vi "fit voltage data to line.vi"(0 "display queues":T1, 1 "disk queues":T1, 5 "crossing time":dbl, 7 "new crossing":bool, 9 "time_buffer":dbl=0.15, 11 "error in (no error)":errorcluster) -> (4 "slope":dbl, 6 "graph":cluster{dbl[], "Best Linear Fit":dbl[]}, 15 "error out":errorcluster)   [LabVIEW 2017]
uses:
  typedefs/queue cluster.ctl
  typedefs/reading queue.ctl
  typedefs/reading.ctl
  typedefs/readingType.ctl
  typedefs/reading1.ctl
  <vilib>/Analysis/6fits.llb/Curve Fitting Criteria.ctl
  <vilib>/Analysis/NI_AALPro.lvlib
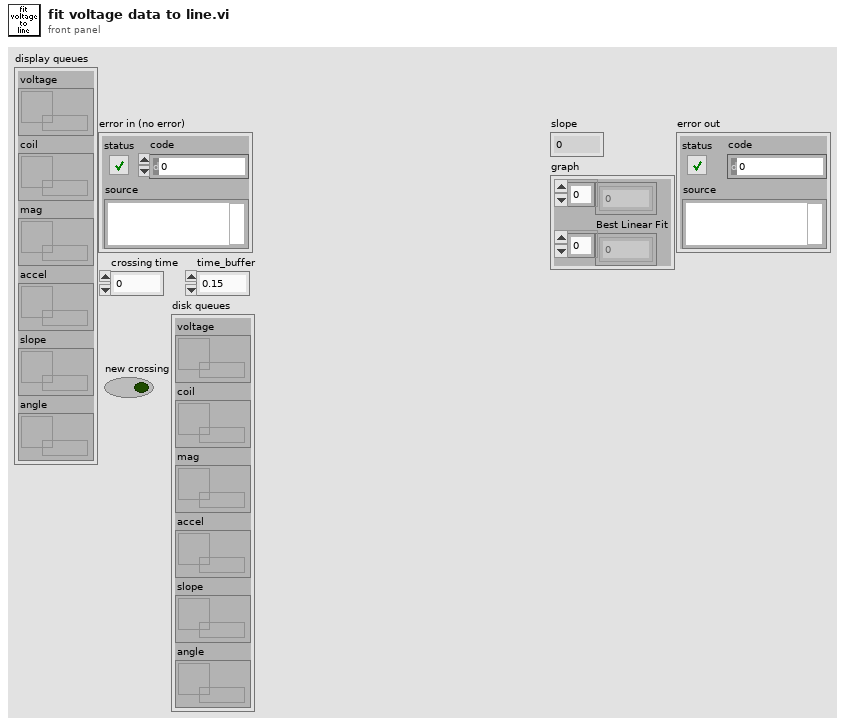
[diagram p1: front panel]
types:
  T1 = typedef "queue cluster.ctl" = cluster{"voltage":T2, "coil":T2, "mag":T2, "accel":T2, "slope":refnum<queue>, "angle":refnum<queue>}
  T2 = typedef "reading queue.ctl" = refnum<queue>
  T3 = typedef "NI_AALPro.lvlib/Curve Fitting Criteria.ctl" = u16
  T4 = typedef "reading.ctl" = cluster{"reading type":T5, "time":fxp<+,48,48>, "x":sgl, "y":sgl, "z":sgl, "XSUM":u8}
  T5 = typedef "readingType.ctl" = enum8{"SYNC", "DETVAL", "COILI", "MAGVEC", "ACCVEC"}
  T6 = cluster{dbl, "slope":dbl, "millisecond timer value":u32}
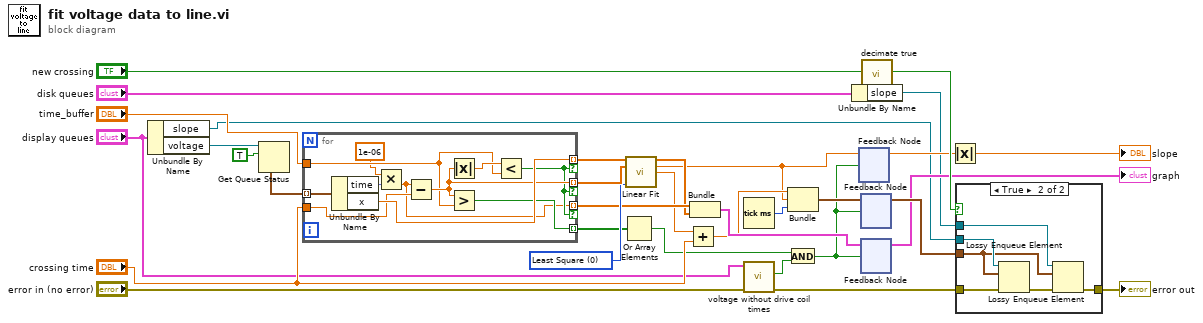
[diagram p0: block diagram]
diagram:
  w30 = T3 0 items=["Least Square", "Least Absolute Residual", "Bisquare"] ("method")
  n1 = Unbundle By Name("display queues") -> ("slope"=w3:refnum<queue>, "voltage"=w7:T2)
  n2 = Get Queue Status(queue=w7, return elements? (F)=TRUE) -> (elements=w5:T4[])  [unwired: 1 in, 7 out]
  n3 = for {
    tunnel: w5 -> [w43] mode=indexing
    tunnel: [w39] -> w31 mode=indexing if=w36
    tunnel: [w42] -> w32 mode=indexing if=w36
    tunnel: "crossing time" -> [w41]
    tunnel: "time_buffer" -> [w38]
    tunnel: [w35] -> w29 mode=indexing if=w36
    tunnel: [w37] -> w18 mode=indexing
    n4 = Unbundle By Name(w43) -> ("time"=w40:fxp<+,48,48>, "x"=w42:sgl)
    n5 = Multiply(x=1e-06, y=w40) -> (x*y=w35:dbl)
    n6 = Subtract(x=w35, y=w41) -> (x-y=w39:dbl)
    n7 = Absolute Value(x=w39) -> (abs(x)=w44:dbl)
    n8 = Greater?(x=w39, y=w38) -> (0:w37:bool)
    n9 = Less?(x=w44, y=w38) -> (x < y?=w36:bool)
  }
  n10 = Or Array Elements(Boolean array=w18) -> (logical OR=w10:bool)
  n11 = call <vilib>:"Linear Fit.vi"("Y"=w32, "X"=w31, "method"=w30) -> ("Best Linear Fit"=w28:dbl[], "slope"=w23:dbl, "intercept"=w26:dbl)  [unwired: 8 in, 2 out]
  n12 = Add(x=w26, y="crossing time") -> (x+y=w24:dbl)
  n13 = Bundle(w29, "Best Linear Fit"=w28) -> (w27:cluster{dbl[], "Best Linear Fit":dbl[]})  [unwired: 1 in]
  n14 = Tick Count (ms)() -> (millisecond timer value=w4:u32)
  n15 = call "voltage without drive coil times.vi"("error in (no error)"="error in (no error)", "display queues"="display queues") -> ("error out"=w12:errorcluster, "not currently in coil veto"=w9:bool)  [unwired: 7 in, 1 out]
  n16 = Bundle(w24, "slope"=w23, "millisecond timer value"=w4) -> (w22:T6)  [unwired: 1 in]
  n17 = And(x=w10, y=w9) -> (x .and. y?=w11:bool)
  n18 = Unbundle By Name("disk queues") -> ("slope"=w1:refnum<queue>)
  n19 = feedback-in #1(w23, w11) -> ()
  n20 = feedback #1() -> (w15:dbl)  [unwired: 1 in]
  n21 = feedback-in #2(w22, w11) -> ()
  n22 = feedback #2() -> (w17:T6)  [unwired: 1 in]
  n23 = feedback-in #3(w27, w11) -> ()
  n24 = feedback #3() -> (→"graph":cluster{dbl[], "Best Linear Fit":dbl[]})  [unwired: 1 in]
  n25 = call "decimate true.vi"("Boolean"="new crossing") -> ("every other true"=w19:bool)  [unwired: 10 in]
  n26 = Absolute Value(x=w15) -> (abs(x)=→"slope":dbl)
  n27 = case shown="True" w19 {
    tunnel: w17 -> [_ w48]
    tunnel: [w45 w46] -> w21
    tunnel: w12 -> [w45 w51]
    tunnel: w3 -> [_ w50]
    tunnel: w1 -> [_ w49]
    frame False {
    }
    frame True {
      n28 = Lossy Enqueue Element(queue=w50, element=w48, error in (no error)=w51) -> (error out=w47:errorcluster)  [unwired: 3 out]
      n29 = Lossy Enqueue Element(queue=w49, element=w48, error in (no error)=w47) -> (error out=w46:errorcluster)  [unwired: 3 out]
    }
  }
  "error out" <- w21
